vi "gentec-SOLO-PE.get Data Sampling Settings.vi"(8 "error in (no error)":errorcluster, 11 "VISA Refnum in":refnum<visa-resource-name>) -> (0 "error out":errorcluster, 1 "Data Samling Settings":T1 {"Time Stamp" items=["Off", "On"]; "Total Duration Unit" items=["Period", "Seconds", "Minutes", "Hours", "Days", "Weeks", "Continuous", "# of Points"]; "Total Duration" max=300 step=1; "Sample Period Unit" items=["Seconds", "Minutes", "Hours", "Days", "Weeks", "Pulses"]; "Sample Rate Unit" items=["per Second", "per Minute", "per Hour", "per Day", "% pulses"]; "Sample Rate" max=300 step=1}, 2 "Error":string, 3 "VISA Refnum out":refnum<visa-resource-name>, 4 "Timeout":bool)   [LabVIEW 2014, in "gentec-SOLO-PE - Driver.lvlib"]
doc: "Gets the Data Sampling Settings."
uses:
  gentec-SOLO-PE - Driver.lvlib
  Type Defs/gentec-SOLO-PE.Data Sampling Settings.ctl
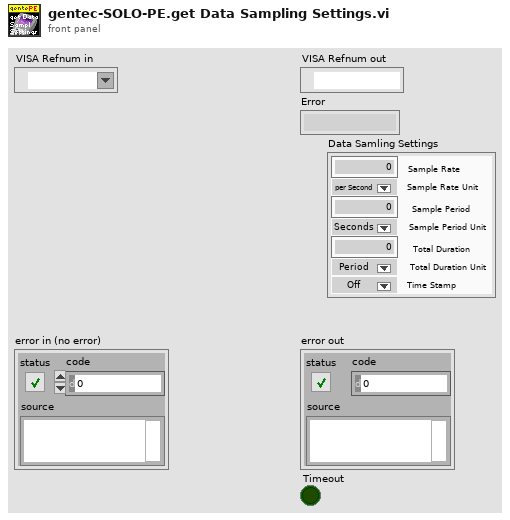
[diagram p1: front panel]
types:
  T1 = typedef "gentec-SOLO-PE - Driver.lvlib/gentec-SOLO-PE.Data Sampling Settings.ctl" = cluster{"Sample Rate":u32, "Sample Rate Unit":u32, "Sample Period":u32, "Sample Period Unit":u32, "Total Duration":u32, "Total Duration Unit":u32, "Time Stamp":u32}
  T2 = cluster{"Return Parameters[0]":u32, "Return Parameters[1]":u32, "Return Parameters[2]":u32, "Return Parameters[3]":u32, "Return Parameters[4]":u32, "Return Parameters[5]":u32, "Return Parameters[6]":u32}
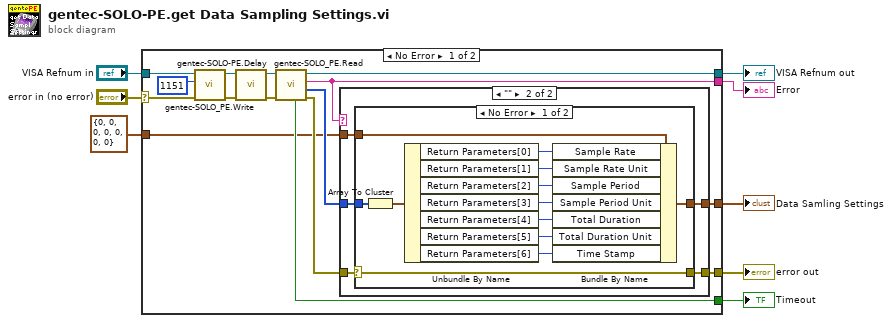
[diagram p0: block diagram]
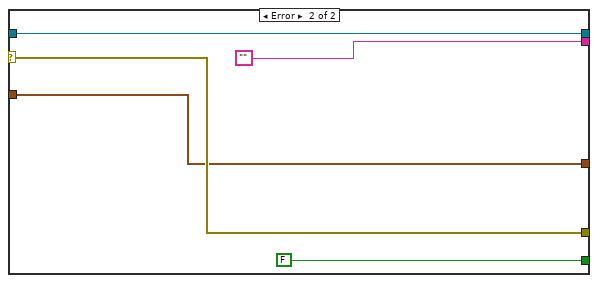
[diagram p4: hidden frame]
diagram:
  n1 = case shown="No Error" "error in (no error)" {
    selector: "error in (no error)" -> [w15 w48]
    tunnel: [w12 w48] -> w8
    tunnel: [w23 w49] -> w7
    tunnel: [w11 ""] -> w6
    tunnel: [w22 FALSE ("Timeout")] -> w5
    tunnel: "VISA Refnum in" -> [w17 w49]
    tunnel: [w10 w45] -> w2
    tunnel: T1 {"Sample Rate"=0, "Sample Rate Unit"=0, "Sample Period"=0, "Sample Period Unit"=0, "Total Duration"=0, "Total Duration Unit"=0, "Time Stamp"=0} ("Configuration") -> [w9 w45]
    frame No Error {
      n2 = call "gentec-SOLO_PE.Write.vi"("error in (no error)"=w15, "Command Handle"=u16 1151, "VISA Refnum in"=w17) -> ("error out"=w20:errorcluster, "VISA Refnum out"=w18:refnum<visa-resource-name>)  [unwired: 7 in]
      n3 = call "gentec-SOLO-PE.Delay.vi"("error in (no error)"=w20, "VISA resource In"=w18) -> ("error out"=w21:errorcluster, "VISA resource Out"=w19:refnum<visa-resource-name>)  [unwired: 4 in]
      n4 = call "gentec-SOLO_PE.Read.vi"("error in (no error)"=w21, "VISA Refnum in"=w19) -> ("error out"=w13:errorcluster, "Return Parameters"=w14:u32[], "Error"=w11:string, "VISA Refnum out"=w23:refnum<visa-resource-name>, "Timeout"=w22:bool)  [unwired: 5 in]
      n5 = case shown="\"\"" w11 {
        tunnel: w14 -> [_ w30]
        tunnel: w13 -> [w25 w29]
        tunnel: [w25 w28] -> w12
        tunnel: w9 -> [w24 w27]
        tunnel: [w24 w26] -> w10
        frame Default {
        }
        frame "" {
          n6 = case shown="No Error" w29 {
            selector: w29 -> [w42 w44]
            tunnel: w30 -> [w35 _]
            tunnel: [w42 w44] -> w28
            tunnel: w27 -> [w37 w43]
            tunnel: [w36 w43] -> w26
            frame No Error {
              n7 = Array To Cluster(array=w35) -> (cluster=w38:T2)
              n8 = Unbundle By Name(w38) -> ("Return Parameters[0]"=w34:u32, "Return Parameters[1]"=w41:u32, "Return Parameters[2]"=w33:u32, "Return Parameters[3]"=w32:u32, "Return Parameters[4]"=w40:u32, "Return Parameters[5]"=w31:u32, "Return Parameters[6]"=w39:u32)
              n9 = Bundle By Name(cluster=w37, "Sample Rate"=w34, "Sample Rate Unit"=w41, "Sample Period"=w33, "Sample Period Unit"=w32, "Total Duration"=w40, "Total Duration Unit"=w31, "Time Stamp"=w39) -> (w36:T1)
            }
            frame Error {
            }
          }
        }
      }
    }
    frame Error {
    }
  }
  "error out" <- w8
  "VISA Refnum out" <- w7
  "Error" <- w6
  "Timeout" <- w5
  "Data Samling Settings" <- w2
